vi "From Veristand Slave To Modbus.vi"(7 "Parameters":T1={"Interface Data"={"Name"="", "Unit ID"=0, "Refresh Rate"=0, "Write Rate"=0, "Write Mode"=enum."Value Change", "Interface Type"=enum."TCP Master", "TCP Settings"={"Address"="", "Port"=0, "Timeout"=0}, "Serial Settings"={"VISA resource name"="", "baud rate"=0, "parity (even)"=0, "flow control (none)"=0, "serial type"=enum."RTU", "Wire Mode"=-1}}, "Modbus Input Groups"=[], "Modbus Output Groups"=[], "error in (no error)"={"status"=FALSE, "code"=0, "source"=""}, "Modbus Input Engine Group Names"=[], "Modbus Output Engine Group Names"=[]} {"Interface Data"."Serial Settings"."Wire Mode" items=["Unknown"=-1, "RS485/Wire4"=0, "RS485/Wire2-EchoDTR"=1, "RS485/Wire2-CtrlDTR"=2, "RS485/Wire2-Auto"=3, "RS232/DTE"=128, "RS232/DCE"=129, "RS232/AUTO"=130]; "Interface Data"."Serial Settings"."parity (even)" items=["None", "Odd", "Even", "Mark", "Space"]; "Interface Data"."Serial Settings"."flow control (none)" items=["None", "XON/XOFF", "RTS/CTS", "XON/XOFF & RTS/CTS", "DTR/DSR", "XON/XOFF & DTR/DSR"]}, 8 "error in (no error)":errorcluster, 10 "Process in":refnum<class "Process.lvclass">, 11 "Modbus Slave in":refnum<class "Modbus Slave.lvclass">) -> ()   [LabVIEW 2020, in "Modbus Master Engine.lvlib"]
uses:
  Modbus Master Engine.lvlib
  <vilib>/NI/NIVS Inline Async API/_VS Inline Async API/Process/Process.lvclass
  <vilib>/NI/NIVS Inline Async API/_Data Access Engine/Data Access Engine/Data Access Engine.lvclass
  <vilib>/NI/NIVS Inline Async API/_Data Access Engine/Data Access Engine/Methods/Write.Lookup.vi
  <vilib>/NI/NIVS Inline Async API/_Data Access Engine/Data Access Engine/Methods/Read.Data.vi
  API/Master/Modbus Master.lvclass
  C:/Users/Administrator/Desktop/GIT/Modbus-Custom-Device-v2/Source/Custom Device Support/API/Modbus API.lvclass
  C:/Users/Administrator/Desktop/GIT/Modbus-Custom-Device-v2/Source/Custom Device Support/API/Master/Modbus Master.lvclass
  API/Slave/Modbus Slave.lvclass
  C:/Users/Administrator/Desktop/GIT/Modbus-Custom-Device-v2/Source/Custom Device Support/API/Slave/Modbus Slave.lvclass
  <vilib>/NI/NIVS Inline Async API/_Data Access Engine/Access Type Classes/Write/Write.lvclass
  <vilib>/NI/NIVS Inline Async API/_Data Access Engine/Access Type Classes/Read/Read.lvclass
  Custom Device/Shared/Controls/Interface Type.ctl
  Custom Device/Shared/Modbus Master Shared.lvlib
  Custom Device/Shared/Controls/Data Model/TCP Settings.ctl
  Custom Device/Shared/Controls/Data Model/Serial Settings.ctl
  Custom Device/System Explorer/SubVIs/Modbus Type.ctl
  Custom Device/Shared/Controls/Data Model/DataType.ctl
  <vilib>/NI VeriStand/Custom Device API/Custom Device Item Ref.ctl
  <vilib>/NI VeriStand/Custom Device API/Custom Device API.lvlib
  Custom Device/Shared/Controls/Data Model/Mapping.ctl
  <vilib>/NI VeriStand/Custom Device API/Custom Device Channel Type.ctl
  Custom Device/Shared/Controls/Data Model/Channel.ctl
  Bulk Data Access.ctl
  Custom Device/Shared/Device Info.ctl
  Custom Device/Shared/Write Mode.ctl
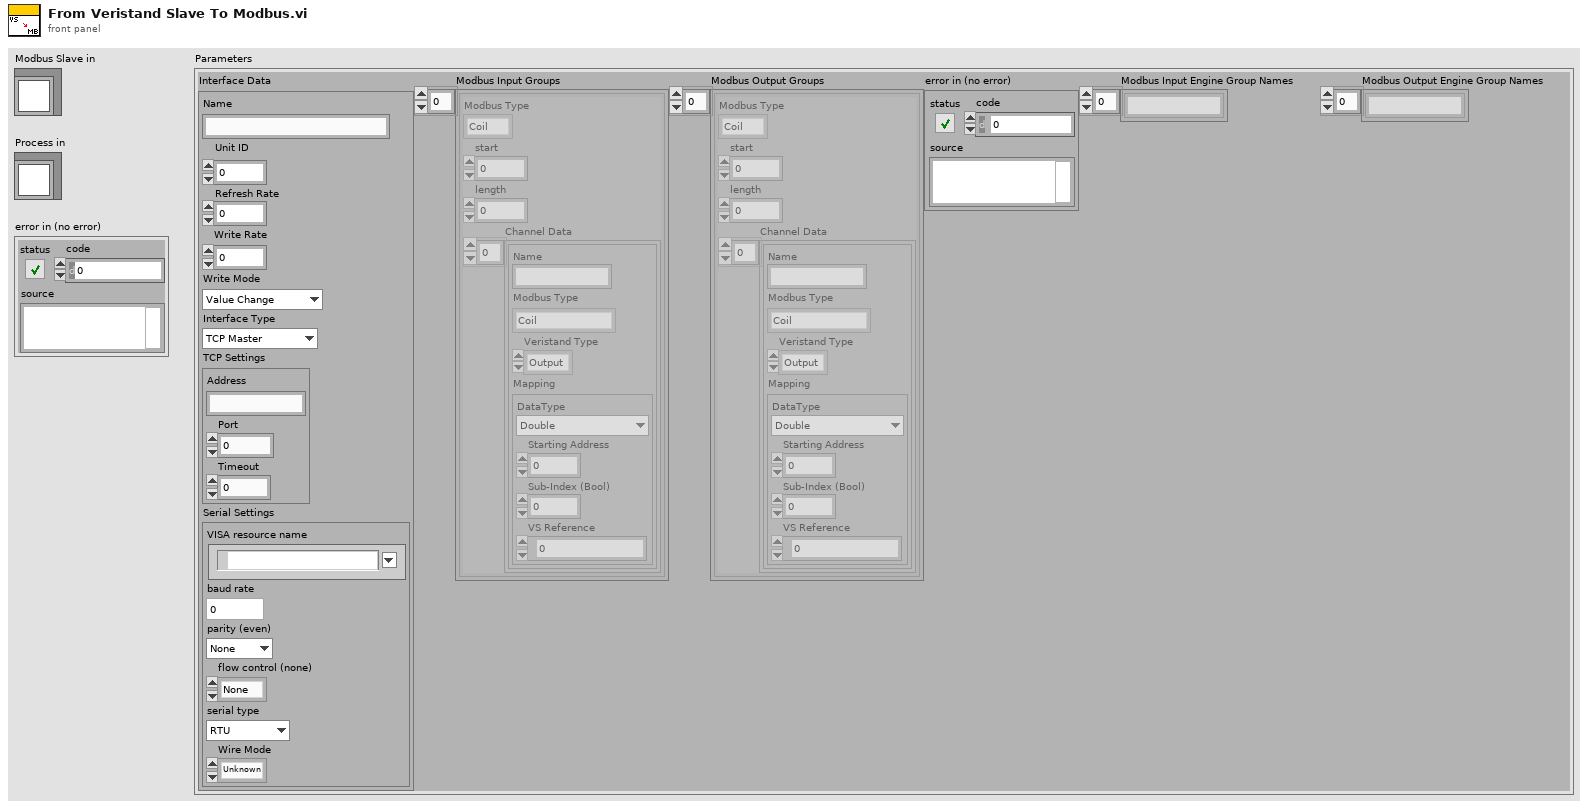
[diagram p1: front panel]
types:
  T1 = typedef "Modbus Master Shared.lvlib/Device Info.ctl" = cluster{"Interface Data":cluster{"Name":string, "Unit ID":u8, "Refresh Rate":i32, "Write Rate":i32, "Write Mode":T2, "Interface Type":T3, "TCP Settings":T4, "Serial Settings":T5}, "Modbus Input Groups":T6[], "Modbus Output Groups":T6[], "error in (no error)":errorcluster, "Modbus Input Engine Group Names":string[], "Modbus Output Engine Group Names":string[]}
  T2 = typedef "Modbus Master Shared.lvlib/Write Mode.ctl" = enum16{"Value Change", "Interval"}
  T3 = typedef "Modbus Master Shared.lvlib/Interface Type.ctl" = enum16{"TCP Master", "Serial Master", "TCP Slave", "Serial Slave"}
  T4 = typedef "Modbus Master Shared.lvlib/TCP Settings.ctl" = cluster{"Address":string, "Port":u16, "Timeout":i32}
  T5 = typedef "Modbus Master Shared.lvlib/Serial Settings.ctl" = cluster{"VISA resource name":refnum<visa-resource-name>, "baud rate":u32, "parity (even)":u16, "flow control (none)":u16, "serial type":enum16{"RTU", "ASCII"}, "Wire Mode":i16}
  T6 = typedef "Modbus Master Shared.lvlib/Bulk Data Access.ctl" = cluster{"Modbus Type":T7, "start":u16, "length":u16, "Channel Data":T8[]}
  T7 = typedef "Modbus Master Shared.lvlib/Modbus Type.ctl" = enum16{"Coil", "Discrete Input", "Holding Register", "Input Register"}
  T8 = typedef "Modbus Master Shared.lvlib/Channel.ctl" = cluster{"Name":string, "Modbus Type":T7, "Veristand Type":T9, "Mapping":T10}
  T9 = typedef "Custom Device API.lvlib/Custom Device Channel Type.ctl" = enum16{"Input", "Output"}
  T10 = typedef "Modbus Master Shared.lvlib/Mapping.ctl" = cluster{"DataType":T11, "Starting Address":u16, "Sub-Index (Bool)":u16, "VS Reference":T12}
  T11 = typedef "Modbus Master Shared.lvlib/DataType.ctl" = enum16{"Double", "Single", "I64", "I32", "I16", "I8", "U64", "U32", "U16", "U8", "Boolean"}
  T12 = typedef "Custom Device API.lvlib/Custom Device Item Ref.ctl" = u64
  T13 = typedef "Data Access Engine.lvlib/Data Access Engine.lvclass/Write.DVR.ctl" = refnum<data-value>
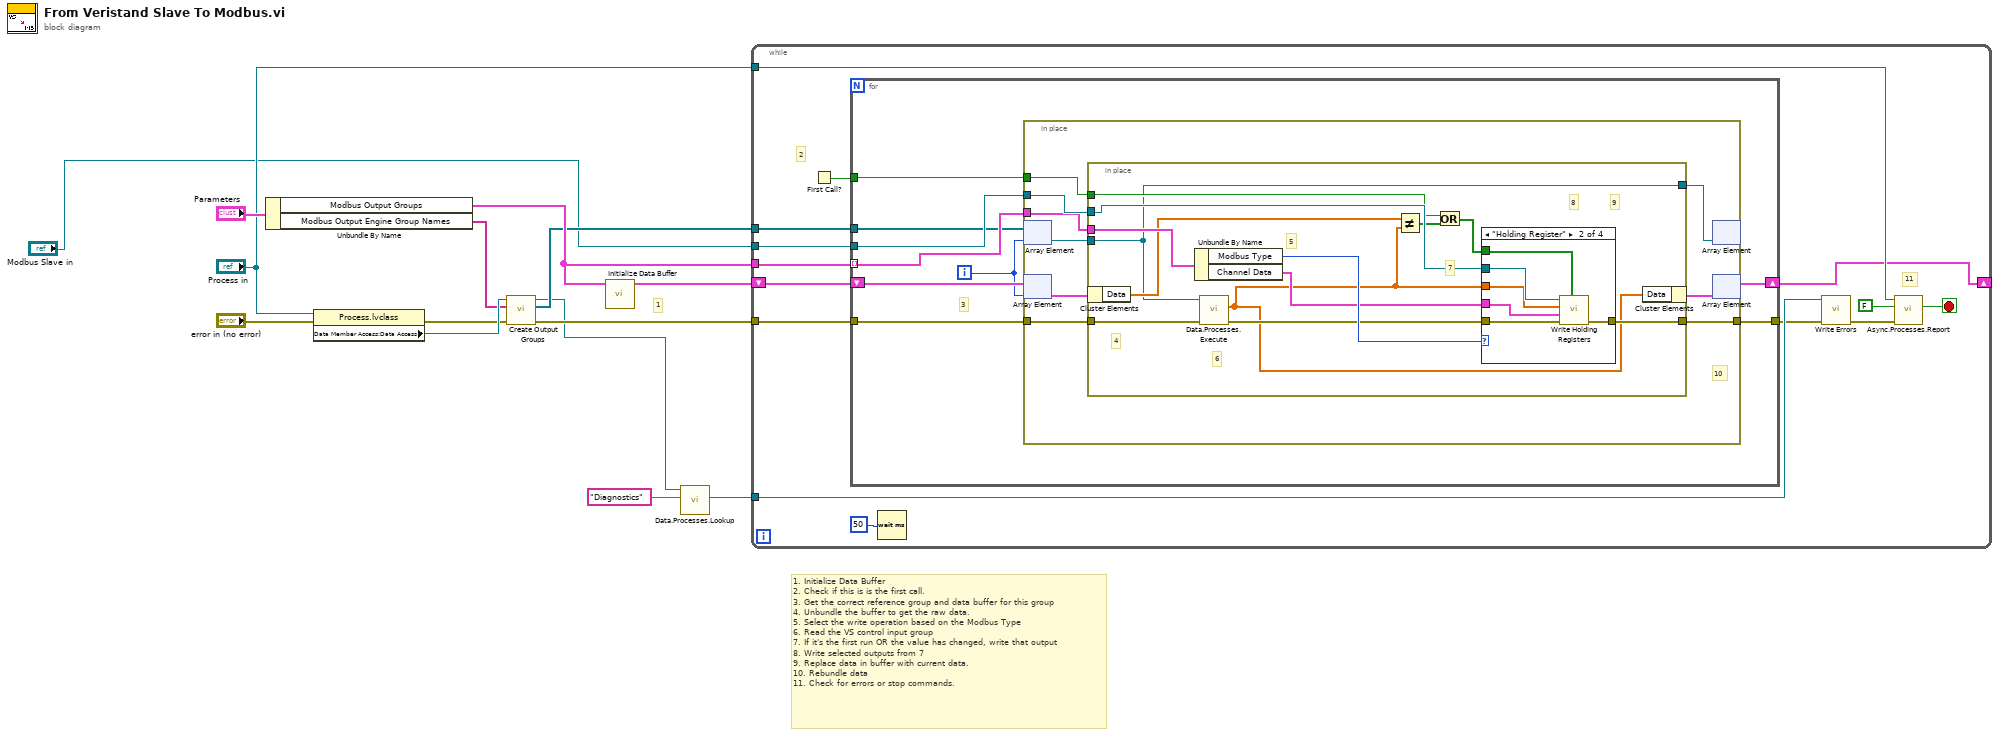
[diagram p0: block diagram]
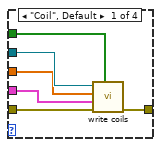
[diagram p2: hidden frame]
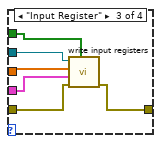
[diagram p3: hidden frame]
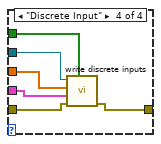
[diagram p4: hidden frame]
diagram:
  # "1"
  # "1. Initialize Data Buffer\n2. Check if this is is the first call.\n3. Get the correct reference group and data buffer for this group\n4. Unbundle the buffer to get the raw data.\n5. Select the write operation based on the Modbus Type\n6. Read the VS control input group\n7. If it's the first run OR the value has changed, write that output\n8. Write selected outputs from 7\n9. Replace data in buffer with current data.\n10. Rebundle data\n11. Check for errors or stop commands."
  n1 = Unbundle By Name("Parameters") -> ("Modbus Output Groups"=w13:T6[], "Modbus Output Engine Group Names"=w9:string[])
  n2 = property class="Process.lvclass"(reference="Process in", error in="error in (no error)") -> (error out=w6:errorcluster, "Data Member Access:Data Access"=w10:refnum<class "Data Access Engine.lvclass">)  [unwired: 1 out]
  n3 = call "Create Output Groups.vi"("error in"=w6, "Input Engine Group Names"=w9, "Data Access Engine in"=w10) -> ("error out"=w5:errorcluster, "Array"=w8:refnum<data-value>[], "Data Access Engine out"=w4:refnum<class "Data Access Engine.lvclass">)  [unwired: 6 in]
  n4 = call "Initialize Data Buffer.vi"("Output Groups"=w13) -> ("Data Buffers"=w12:cluster{"Data":dbl[]}[])  [unwired: 10 in]
  n5 = call-poly <vilib>:"Data.Processes.Lookup.vi"("Name"="Diagnostics", "Data Access API in"=w4) -> ("Ref"=w2:T13)  [unwired: 6 in, 3 out]
  n6 = while {
    tunnel: "Process in" -> [w28]
    tunnel: w8 -> [w25]
    tunnel: w13 -> [w27]
    tunnel: "Modbus Slave in" -> [w26]
    tunnel: w5 -> [w24]
    shift-right: [w21] -> _
    shift-left: w12 -> [w22]
    tunnel: w2 -> [w17]
    stop <- w23 stop-if-true
    # "11"
    # "2"
    n7 = First Call?() -> (First Call?: T/F=w18:bool)
    n8 = for {
      tunnel: w27 -> [w36] mode=indexing
      tunnel: w26 -> [w37]
      tunnel: w25 -> [w31]
      tunnel: w24 -> [w35]
      tunnel: [w34] -> w16
      shift-right: [w32] -> w21
      shift-left: w22 -> [w33]
      tunnel: w18 -> [w29]
      i -> [w30]
      # "3"
      n9 = in-place {
        in-place-border: w37 -> [w46]
        in-place-border: w36 -> [w45]
        in-place-border: w35 -> [w44]
        in-place-border: [w43] -> w34
        in-place-border: w29 -> [w38]
        # "10"
        n10 = in-place-array #1(w31, w30) -> (w40:refnum<data-value>)
        n11 = in-place-array #2(w33, w30) -> (w42:cluster{"Data":dbl[]})
        n12 = in-place {
          in-place-border: w46 -> [w59]
          in-place-border: w45 -> [w58]
          in-place-border: w44 -> [w50]
          in-place-border: [w57] -> w43
          in-place-border: w40 -> [w51]
          in-place-border: [w51] -> w39
          in-place-border: w38 -> [w52]
          # "8"
          # "5"
          # "7"
          # "6"
          # "9"
          # "4"
          n13 = in-place-cluster #3(w42) -> ("Data"=w53:dbl[])
          n14 = Unbundle By Name(w58) -> ("Modbus Type"=w56:T7, "Channel Data"=w55:T8[])
          n15 = call-poly <vilib>:"Data.Processes.Execute.vi"("error in (no error)"=w50, "Ref"=w51) -> ("error out"=w49:errorcluster, "Values"=w47:dbl[])  [unwired: 7 in, 1 out]
          n16 = Not Equal?(x=w53, y=w47) -> (x != y?=w54:bool[])
          n17 = Or(x=w52, y=w54) -> (x .or. y?=w48:bool[])
          n18 = case shown="\"Holding Register\"" w56 {
            tunnel: w59 -> [w65 w71 w77 w83]
            tunnel: [w64 w70 w72 w82] -> w57
            tunnel: w49 -> [w63 w69 w73 w81]
            tunnel: w55 -> [w60 w68 w74 w80]
            tunnel: w48 -> [w62 w67 w76 w78]
            tunnel: w47 -> [w61 w66 w75 w79]
            frame "Coil", Default {
              n19 = call "write coils.vi"("Write Mask"=w62, "error in (no error)"=w63, "Channel Data"=w60, "Values"=w61, "Modbus API.lvlibp:Modbus API"=w65) -> ("error out"=w64:errorcluster)  [unwired: 6 in]
            }
            frame "Holding Register" {
              n20 = call "Write Holding Registers.vi"("Regs to Write"=w67, "error in (no error)"=w69, "Channel Data"=w68, "Values"=w66, "Modbus API.lvlibp:Modbus API"=w71) -> ("error out"=w70:errorcluster)  [unwired: 6 in]
            }
            frame "Input Register" {
              n21 = call "write input registers.vi"("Regs to Write"=w76, "error in (no error)"=w73, "Channel Data"=w74, "Values"=w75, "Modbus slave in"=w77) -> ("error out"=w72:errorcluster)  [unwired: 6 in]
            }
            frame "Discrete Input" {
              n22 = call "write discrete inputs.vi"("Array"=w78, "error in (no error)"=w81, "Channel Data"=w80, "Values"=w79, "Modbus Slave In"=w83) -> ("error out"=w82:errorcluster)  [unwired: 6 in]
            }
          }
          n23 = in-place-cluster #3("Data"=w47) -> (w41:cluster{"Data":dbl[]})
        }
        n24 = in-place-array #1(w39) -> ()  [unwired: 2 out]
        n25 = in-place-array #2(w41) -> (w32:cluster{"Data":dbl[]}[])  [unwired: 1 out]
      }
    }
    n26 = Wait (ms)(milliseconds to wait=u32 50) -> ()  [unwired: 1 out]
    n27 = call "Write Errors.vi"("error in (no error)"=w16, "Data Value Reference in"=w17) -> ("error out"=w15:errorcluster)  [unwired: 9 in]
    n28 = call <vilib>:"Async.Processes.Report.vi"("Error"=w15, "Stop Async on Error?"=FALSE ("Stop on Error?"), "Process in"=w28) -> ("Stop"=w23:bool)  [unwired: 7 in, 1 out]
  }
